vi "append_to_CSV.vi"(8 "error in (no error)":errorcluster, 10 "text":string, 11 "file_path":path) -> (0 "error out":errorcluster)   [LabVIEW 2018]
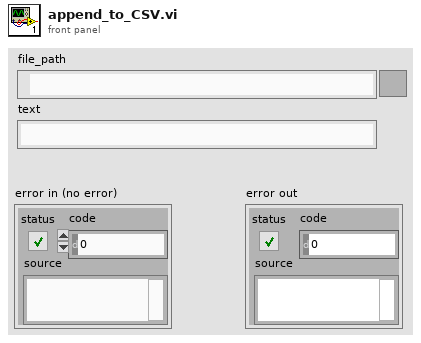
[diagram p1: front panel]
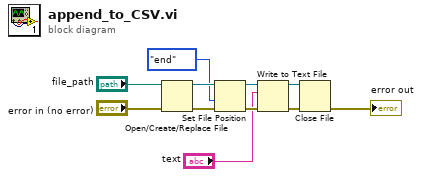
[diagram p0: block diagram]
diagram:
  n1 = Open/Create/Replace File(file path (use dialog)="file_path", error in="error in (no error)") -> (refnum out=w10:refnum<file>, error out=w7:errorcluster)  [unwired: 4 in, 1 out]
  n2 = Set File Position(refnum=w10, from (0:start)=enum16{"start", "end", "current"}."end", error in=w7) -> (refnum out=w9:refnum<file>, error out=w6:errorcluster)  [unwired: 1 in]
  n3 = Write to Text File(file (use dialog)=w9, text="text", error in=w6) -> (refnum out=w8:refnum<file>, error out=w5:errorcluster)  [unwired: 1 in, 1 out]
  n4 = Close File(refnum=w8, error in=w5) -> (error out=→"error out":errorcluster)  [unwired: 1 out]
